vi "Sandbox.vi"() -> ()   [LabVIEW 2019, in "FPGA_Concrete.lvclass"]
uses:
  FPGA_Concrete.lvclass
  <vilib>/Platform/TimedLoop/XDataNode/timing_clust.ctl
  <vilib>/Platform/TimedLoop/XDataNode/nitl_modes.ctl
  <vilib>/Platform/TimedLoop/XDataNode/wakeup.ctl
  692d18c9-0166-474d-9980-2d6284fd9cd3.vi
  <vilib>/platform/TimedLoop/XDataNode/XDataNode.xnode
  <vilib>/Platform/TimedLoop/XDataNode/XDNodeRunTimeDep.lvlib
panel:
  out "AIs":dbl[](array[numeric]) format="%#.6f"
  in  "DOs 2":bool[](array[boolean])
  out "AOs":dbl[](array[numeric])
  out "error out 2":errorcluster
  out "DOs":bool[](array[boolean])
  out "appended array":bool[](array[boolean])
  in  "index DI":i32
  out "Iteration Duration":i64
  out "Waveform Chart":dbl[][](graph)
  in  "Set DO":bool
  in  "Value AO":dbl
  in  "Indx AO":i32
  out "DIs":bool[](array[boolean])
  out "data valid":bool
  in  "stop":bool
  out "error out":errorcluster
  # "0"
  # "4"
  # "8"
  # "12"
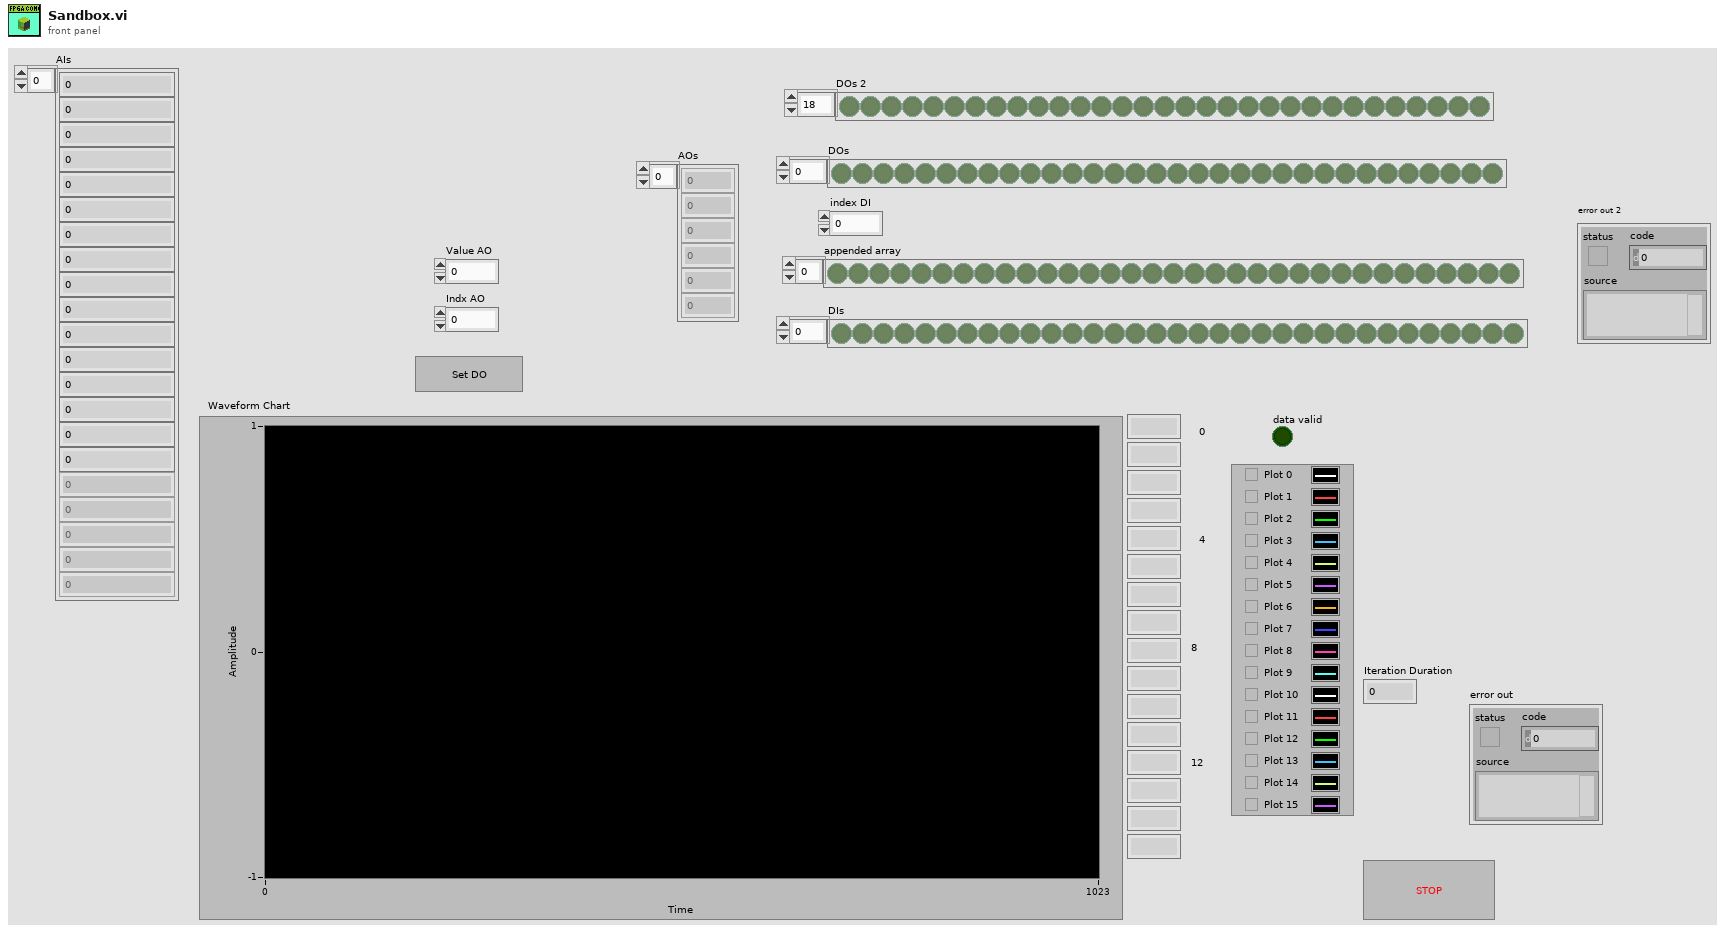
[diagram p1: front panel]
types:
  T1 = typedef "XDNodeRunTimeDep.lvlib/timing_clust.ctl" = cluster{"Expected End [f-1]":u64, "Actual End [f-1]":u64, "Finished Late? [f-1]":bool, "Expected End [i-1]":u64, "Actual End [i-1]":u64, "Finished Late? [i-1]":bool, "Expected Start [i]":u64, "Actual Start [i]":u64, "Expected Start [f]":u64, "Actual Start [f]":u64, "Source Name":string, "Structure Name":string, "Period":i64, "Deadline":i64, "Offset":i64, "Start":i64, "Priority":i32, "Timeout":i32, "Mode":T2, "Wakeup Reason":T3, "Error":errorcluster, "Source Type":string, "Secondary Source Type":string, "Global End Time":u64, "Global Start Time":u64, "Frame Duration":u64, "Iteration Duration":u64, "Assigned CPU":i32, "I/O Scan Engine Mode":u32}
  T2 = typedef "XDNodeRunTimeDep.lvlib/nitl_modes.ctl" = enum32{"No Change", "Process missed periods, maintain original phase", "Discard missed periods, maintain original phase", "Process missed periods, ignore original phase", "Discard missed periods, ignore original phase"}
  T3 = typedef "XDNodeRunTimeDep.lvlib/wakeup.ctl" = enum32{"Normal", "Aborted", "Asynchronous wakeup", "Timing source error", "Timed loop error", "Timeout"}
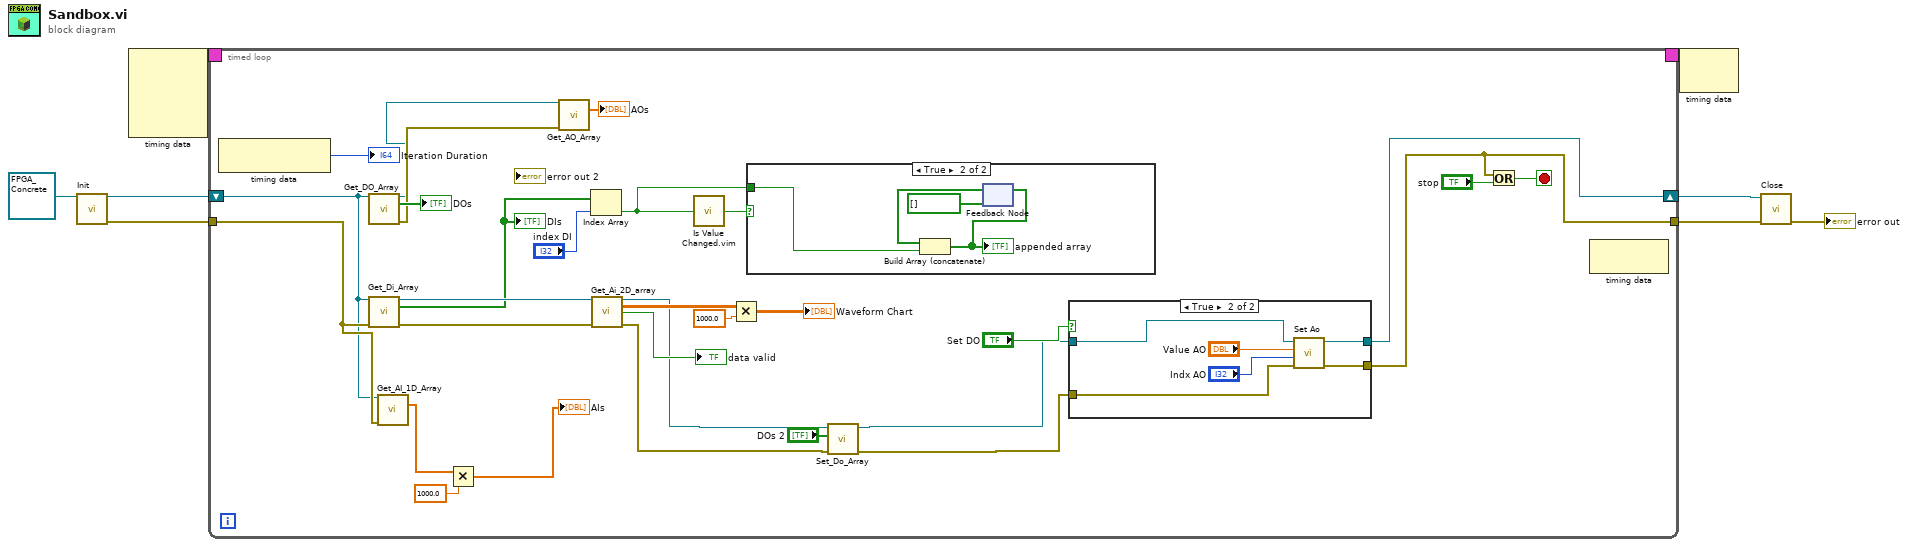
[diagram p0: block diagram]
diagram:
  n1 = call-dynamic "Init.vi"("reference in"=refnum<class "FPGA_Concrete.lvclass"> refnum) -> ("reference out"=w7:refnum<class "FPGA_Concrete.lvclass">, "error out"=w2:errorcluster)  [unwired: 13 in]
  n2 = node-c288() -> (w4:T1)  [unwired: 4 in]
  n3 = timed-loop {
    timing: w4 -> [_]
    timing-out: [_] -> w3
    shift-right: [w37] -> w6
    shift-left: w7 -> [w12]
    tunnel: w2 -> [w13]
    tunnel: [w33] -> w1
    stop <- w34 stop-if-true
    n4 = node-c288() -> (→"Iteration Duration":i64)  [unwired: 1 in]
    n5 = call-dynamic "Get_DO_Array.vi"("reference in"=w12) -> ("reference out"=w20:refnum<class "FPGA_Concrete.lvclass">, "DOs"=→"DOs":bool[], "error out"=w21:errorcluster)  [unwired: 12 in]
    n6 = call-dynamic "Get_Di_Array.vi"("reference in"=w12, "error in (no error)"=w13) -> ("reference out"=w38:refnum<class "FPGA_Concrete.lvclass">, "DIs"=w29:bool[], "error out"=w36:errorcluster)  [unwired: 11 in]
    "DIs" <- w29
    n7 = call-dynamic "Get_AI_1D_Array.vi"("reference in"=w12, "error in (no error)"=w13) -> ("AIs"=w11:dbl[])  [unwired: 11 in, 2 out]
    n8 = Multiply(x=w11, y=1000.0) -> (x*y=→"AIs":dbl[])
    n9 = call-dynamic "Get_AO_Array.vi"("reference in"=w20, "error in (no error)"=w21) -> ("AOs"=→"AOs":dbl[])  [unwired: 11 in, 2 out]
    n10 = Index Array(array=w29, index="index DI") -> (element=w26:bool)
    n11 = call-dynamic "Get_Ai_2D_array.vi"("reference in"=w38, "error in (no error)"=w36) -> ("reference out"=w18:refnum<class "FPGA_Concrete.lvclass">, "AIs"=w31:dbl[][], "data valid"=→"data valid":bool, "error out"=w17:errorcluster)  [unwired: 10 in]
    n12 = call "Is Value Changed.vim"("value"=w26) -> ("changed or first call?"=w27:bool)
    n13 = Multiply(x=w31, y=1000.0) -> (x*y=→"Waveform Chart":dbl[][])
    n14 = case shown="True" w27 {
      tunnel: w26 -> [_ w42]
      frame False {
      }
      frame True {
        n15 = feedback #1(bool[] []) -> (w40:bool[])
        n16 = Build Array (concatenate)(w40, w42) -> (w41:bool[])
        "appended array" <- w41
        n17 = feedback-in #1(w41) -> ()
      }
    }
    n18 = call-dynamic "Set_Do_Array.vi"("error in (no error)"=w17, "DOs"="DOs 2", "reference in"=w18) -> ("error out"=w16:errorcluster, "reference out"=w15:refnum<class "FPGA_Concrete.lvclass">)  [unwired: 7 in]
    n19 = case shown="True" "Set DO" {
      tunnel: w15 -> [w44 w50]
      tunnel: [w44 w49] -> w37
      tunnel: w16 -> [w43 w48]
      tunnel: [w43 w47] -> w33
      frame False {
      }
      frame True {
        n20 = call-dynamic "Set Ao.vi"("error in (no error)"=w48, "Indx"="Indx AO", "Value"="Value AO", "FPGA_Concrete in"=w50) -> ("error out"=w47:errorcluster, "FPGA_Concrete out"=w49:refnum<class "FPGA_Concrete.lvclass">)  [unwired: 6 in]
      }
    }
    n21 = Or(x=w33, y="stop") -> (x .or. y?=w34:bool)
    n22 = node-c288() -> ()  [unwired: 1 in, 1 out]
  }
  n23 = node-c288(w3) -> ()  [unwired: 1 out]
  n24 = call-dynamic "Close.vi"("error in (no error)"=w1, "FPGA_Concrete in"=w6) -> ("error out"=→"error out":errorcluster)  [unwired: 8 in, 1 out]
